vi "sub_Control_Save_or_Load.vi"(5 "Enum":enum16{"Save", "Load"}(ring), 8 "error in":errorcluster, 10 "Array":refnum<vi>[](array[refnum]), 11 "File Path":path) -> (0 "error out":errorcluster)   [LabVIEW 2023]
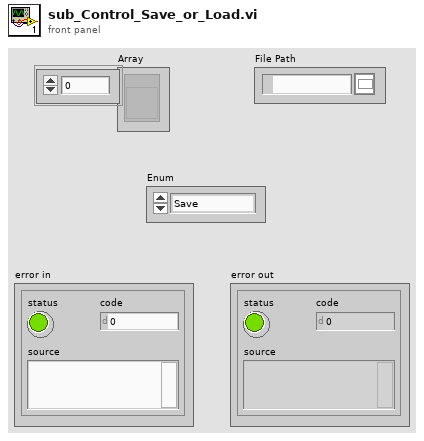
[diagram p1: front panel]
types:
  T1 = enum16{"open", "replace", "create", "open or create", "replace or create", "replace or create with confirmation"}
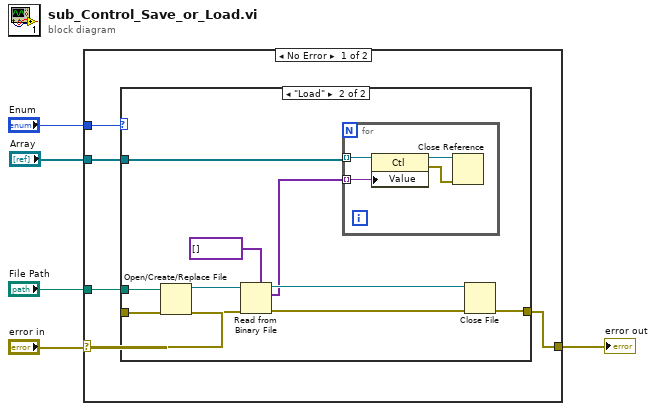
[diagram p0: block diagram]
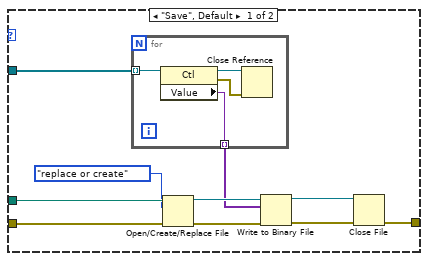
[diagram p2: hidden frame]
diagram:
  n1 = case shown="No Error" "error in" {
    selector: "error in" -> [w8 w39]
    tunnel: [w7 w39] -> w4
    tunnel: "Enum" -> [w10 _]
    tunnel: "File Path" -> [w9 _]
    tunnel: "Array" -> [w6 _]
    frame No Error {
      n2 = case shown="\"Load\"" w10 {
        tunnel: w9 -> [w20 w29]
        tunnel: w8 -> [w17 w28]
        tunnel: [w14 w25] -> w7
        tunnel: w6 -> [w13 w30]
        frame "Save", Default {
          n3 = for {
            tunnel: w13 -> [w24] mode=indexing
            tunnel: [w21] -> w12 mode=indexing
            n4 = property class="Ctl"(reference=w24) -> (reference out=w22:refnum<vi>, error out=w23:errorcluster, "Value"=w21:variant)  [unwired: 1 in]
            n5 = Close Reference(reference=w22, error in (no error)=w23) -> ()  [unwired: 1 out]
          }
          n6 = Open/Create/Replace File(file path (use dialog)=w20, error in=w17, operation (0:open)=T1."replace or create") -> (refnum out=w19:refnum<file>, error out=w16:errorcluster)  [unwired: 3 in, 1 out]
          n7 = Write to Binary File(file (use dialog)=w19, data=w12, error in=w16) -> (refnum out=w18:refnum<file>, error out=w15:errorcluster)  [unwired: 3 in, 1 out]
          n8 = Close File(refnum=w18, error in=w15) -> (error out=w14:errorcluster)  [unwired: 1 out]
        }
        frame "Load" {
          n9 = Open/Create/Replace File(file path (use dialog)=w29, error in=w28) -> (refnum out=w34:refnum<file>, error out=w32:errorcluster)  [unwired: 4 in, 1 out]
          n10 = Read from Binary File(5:variant[] [], 8:w32, 11:w34) -> (0:w31:errorcluster, 2:w27:variant[], 3:w33:refnum<file>)  [unwired: 3 in, 1 out]
          n11 = for {
            tunnel: w30 -> [w38] mode=indexing
            tunnel: w27 -> [w35] mode=indexing
            n12 = property class="Ctl"(reference=w38, "Value"=w35) -> (reference out=w36:refnum<vi>, error out=w37:errorcluster)  [unwired: 1 in]
            n13 = Close Reference(reference=w36, error in (no error)=w37) -> ()  [unwired: 1 out]
          }
          n14 = Close File(refnum=w33, error in=w31) -> (error out=w25:errorcluster)  [unwired: 1 out]
        }
      }
    }
    frame Error {
    }
  }
  "error out" <- w4
